vi "Detect Image Pipleline.vi"(8 "error in (no error)":errorcluster, 11 "Microscope_RM21 in":refnum<class "Microscope_RM21.lvclass">) -> (0 "error out":errorcluster, 3 "Microscope_RM21 out":refnum<class "Microscope_RM21.lvclass">)   [LabVIEW 2020, in "Microscope_RM21.lvlib" / "Microscope_RM21.lvclass"]
uses:
  Microscope_RM21.lvclass
  Logic Layer/SingleParticleTracking/SingleParticleTracking/SingleParticleTracking.lvclass
  D:/Daguan/Development/MMicroscopyAF/Model/Logic Layer/ImagePipeline/ImagePipeline.lvclass
  Logic Layer/ImagePipeline Messages/SetUpImageBuffer Msg/SetUpImageBuffer Msg.lvclass/SetUpImageBuffer Msg.ctl
  <vilib>/ActorFramework/Message Enqueuer/Message Enqueuer.lvclass/Message Enqueuer.ctl
  <vilib>/ActorFramework/Message Enqueuer/Enqueue.vi
  Logic Layer/ImagePipeline Messages/SetUpImageBuffer Msg/SetUpImageBuffer Msg.lvclass
  C:/Program Files/National Instruments/LabVIEW 2020/vi.lib/ActorFramework/Message/Message.lvclass
  <vilib>/ActorFramework/Message Priority Queue/Priority Enqueue.vi
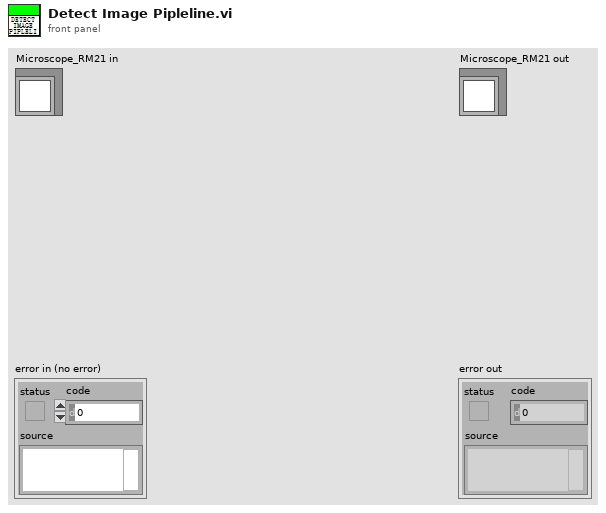
[diagram p1: front panel]
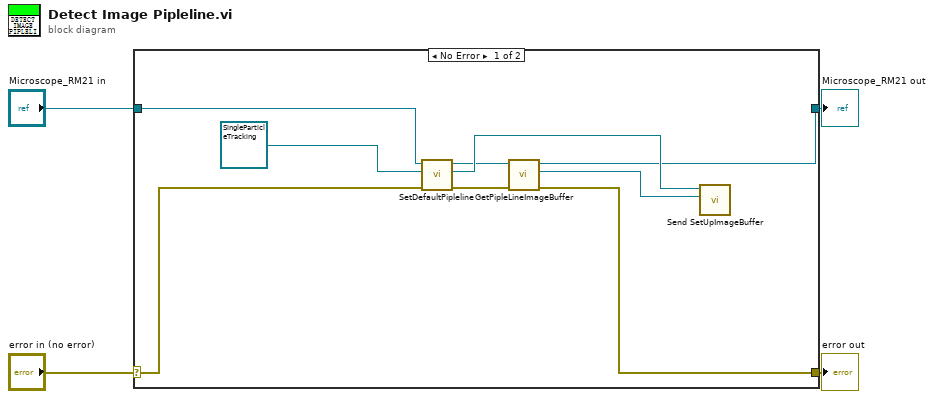
[diagram p0: block diagram]
diagram:
  n1 = case shown="No Error" "error in (no error)" {
    selector: "error in (no error)" -> [w12 w15]
    tunnel: [w5 w15] -> w3
    tunnel: [w8 w14] -> w1
    tunnel: "Microscope_RM21 in" -> [w13 w14]
    frame No Error {
      n2 = call-dynamic "SetDefaultPipleline.vi"("error in (no error)"=w12, "Image Pipleline In"=refnum<class "SingleParticleTracking.lvclass"> refnum ("SingleParticleTracking.lvlib:SingleParticleTracking.lvclass"), "Microscope in"=w13) -> ("error out"=w6:errorcluster, "Enqueuer"=w10:refnum<class "Message Enqueuer.lvclass">, "Microscope out"=w9:refnum<class "Microscope_RM21.lvclass">)  [unwired: 6 in]
      n3 = call-dynamic "GetPipleLineImageBuffer.vi"("error in (no error)"=w6, "Microscope in"=w9) -> ("error out"=w5:errorcluster, "PiplelineImageBuffers"=w7:refnum<queue>, "Microscope out"=w8:refnum<class "Microscope_RM21.lvclass">)  [unwired: 7 in]
      n4 = call "Send SetUpImageBuffer.vi"("ImageBuffers"=w7, "Message Enqueuer"=w10) -> ()  [unwired: 8 in, 2 out]
    }
    frame Error {
    }
  }
  "error out" <- w3
  "Microscope_RM21 out" <- w1
